vi "gate width to percent.vi"(2 "Trigger Freq":dbl[unit], 3 "Gate width":dbl[unit]) -> (1 "Gate %":dbl)   [LabVIEW 2011]
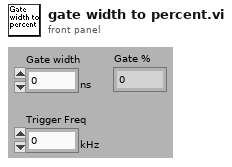
[diagram p1: front panel]
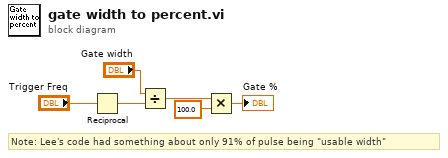
[diagram p0: block diagram]
diagram:
  # "Note: Lee's code had something about only 91% of pulse being \"usable width\""
  n1 = Reciprocal(x="Trigger Freq") -> (1/x=w3:dbl[unit])
  n2 = Divide(x="Gate width", y=w3) -> (x/y=w2:dbl)
  n3 = Multiply(x=w2, y=100.0) -> (x*y=→"Gate %":dbl)
